vi "StateMachineDAQ-MultiChannel.vi"() -> ()   [LabVIEW 2014]
doc: "Use this template to build a user interface event handler design pattern. Use this pattern for dialog boxes and other user interfaces. You also can create and execute user-defined events that the VI can handle the same way as user interface events."
uses:
  subVIs/StateMachineDAQState.ctl
  <vilib>/Utility/error.llb/DialogType.ctl
  <vilib>/DAQmx/create/channels.llb/DAQmx Create Channel (AI-Voltage-Basic).vi
  <vilib>/DAQmx/configure/timing.llb/DAQmx Timing (Sample Clock).vi
  <vilib>/DAQmx/read.llb/DAQmx Read (Analog 1D Wfm NChan NSamp).vi
  <resource>/objmgr/daqmx.rc
panel:
  in  "File Path":path
  in  "Acquire Data":bool
  in  "Log Data":bool
  in  "File Comment":string
  in  "DAQ Parameters":T1={"rate"=1000.0, "read period"=0.5, "Channels"=[]} {"Channels"."minimum value" format="%0.2f"; "Channels"."maximum value" format="%0.2f"; "read period" format="%0.2f"; "rate" format="%0.2f"}
  out "Waveform Chart":waveform(dbl)[](graph)
  in  "quit":bool
  # "Hz"
  # "s"
  # "V"
  # "V"
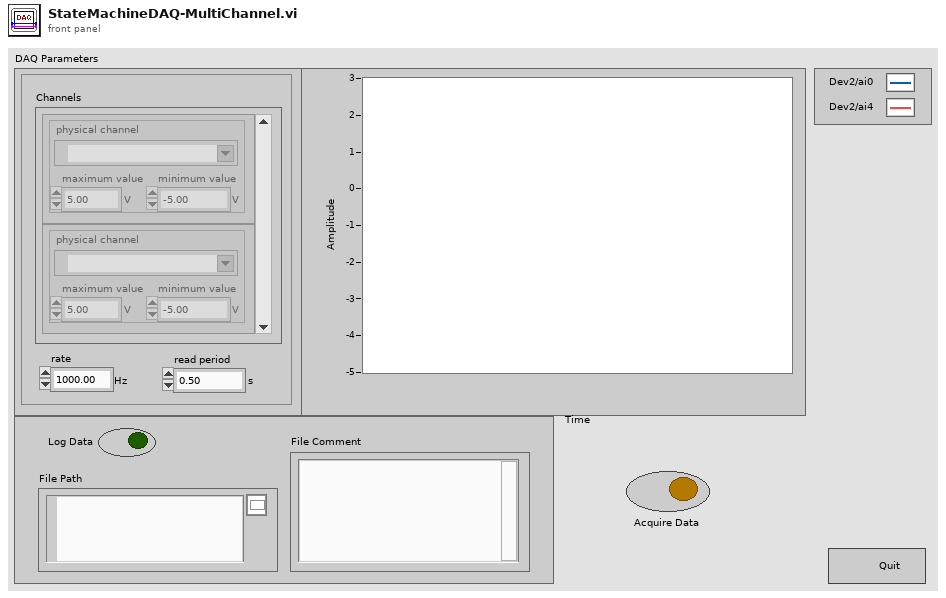
[diagram p1: front panel]
types:
  T1 = cluster{"rate":dbl, "read period":dbl, "Channels":cluster{"physical channel":tag, "maximum value":dbl, "minimum value":dbl}[]}
  T2 = typedef "StateMachineDAQState.ctl" = enum16{"Init", "Idle", "CheckError", "Finalize", "ConfigDAQ", "StartDAQ", "AcquireAndLog", "StopDAQ", "ClearDAQ", "OpenFile", "CloseFile", "Process 1"}
  T3 = typedef "DialogType.ctl" = u16
  T4 = cluster{"physical channel":tag, "maximum value":dbl, "minimum value":dbl}[]
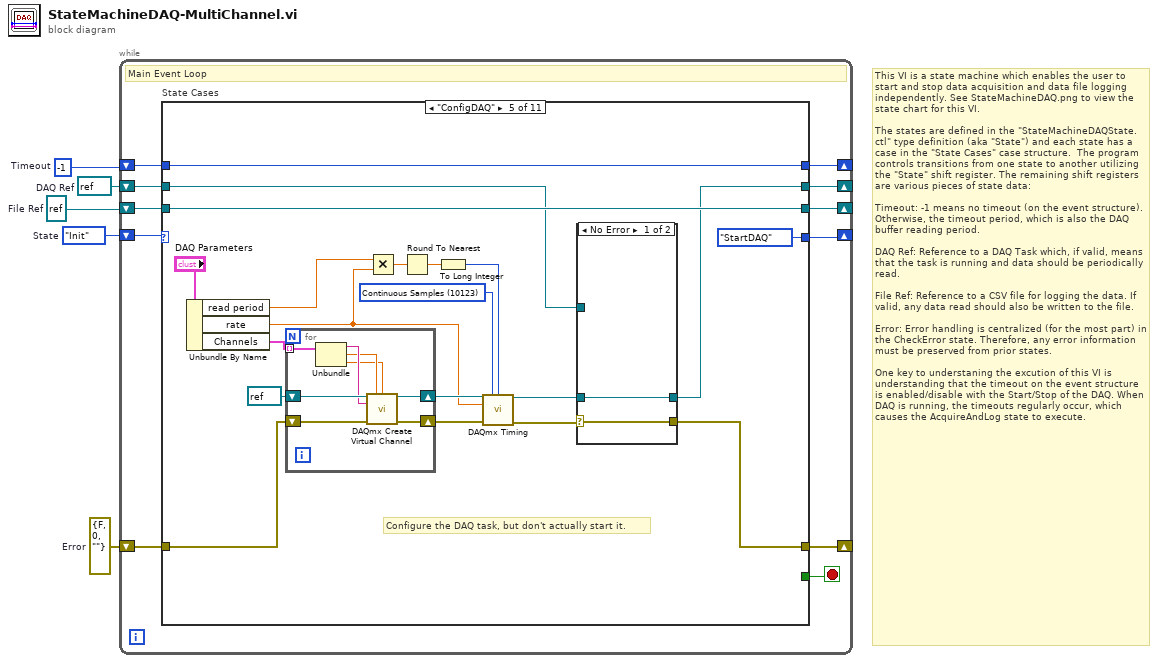
[diagram p0: block diagram]
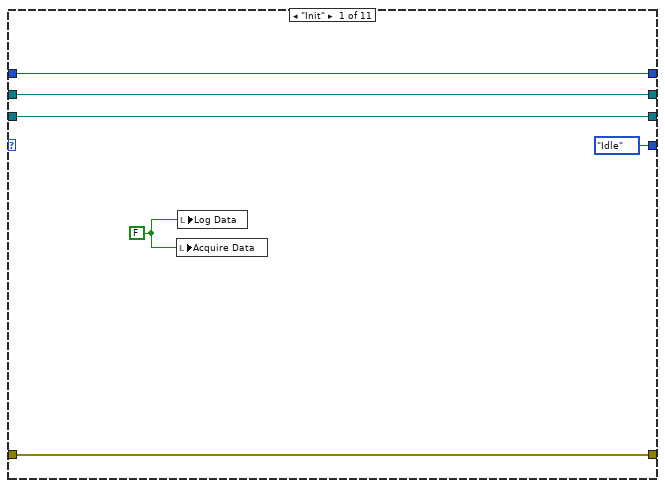
[diagram p2: hidden frame]
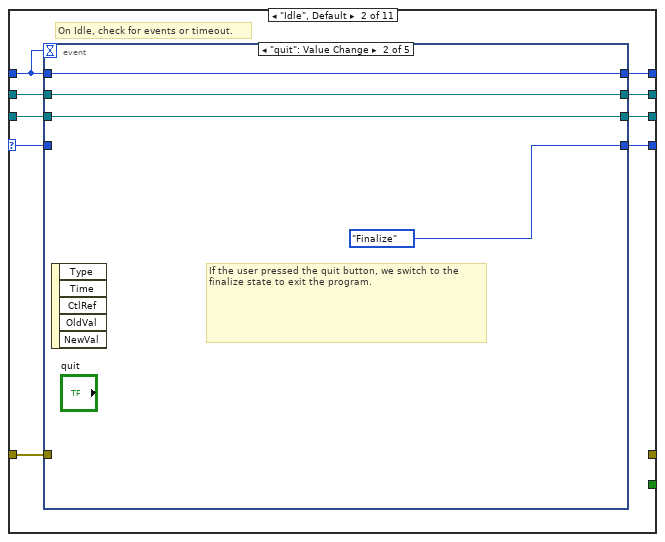
[diagram p3: hidden frame]
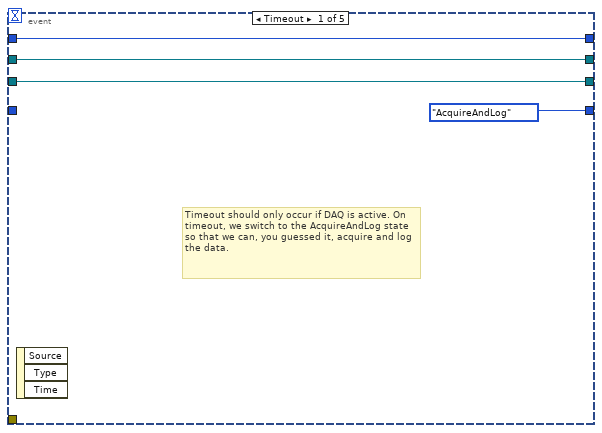
[diagram p4: hidden frame]
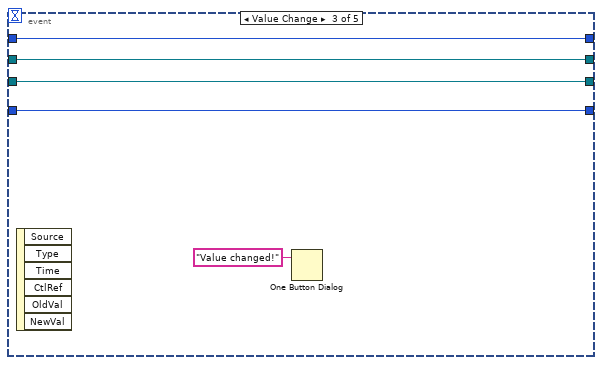
[diagram p5: hidden frame]
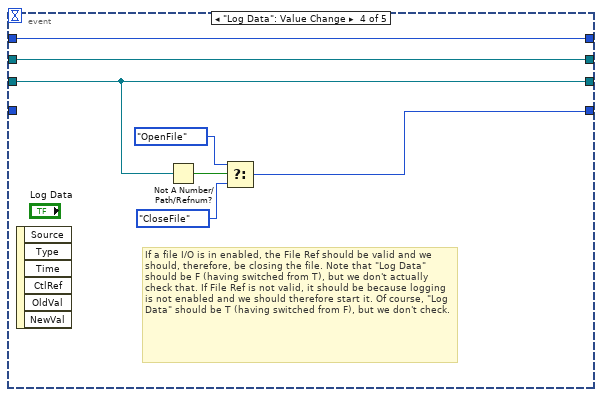
[diagram p6: hidden frame]
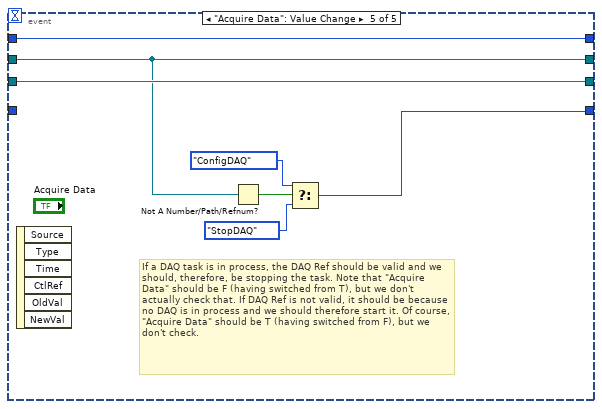
[diagram p7: hidden frame]
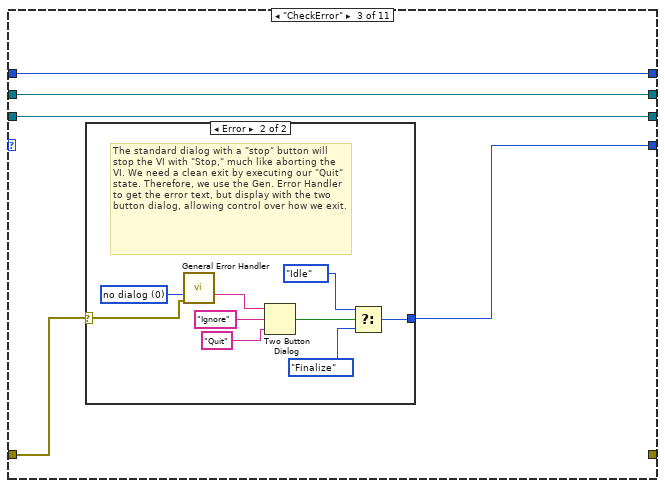
[diagram p8: hidden frame]
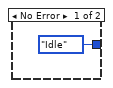
[diagram p9: hidden frame]
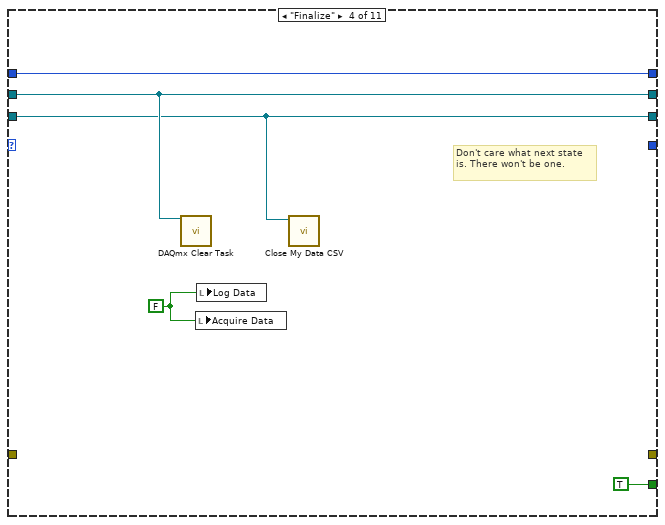
[diagram p10: hidden frame]
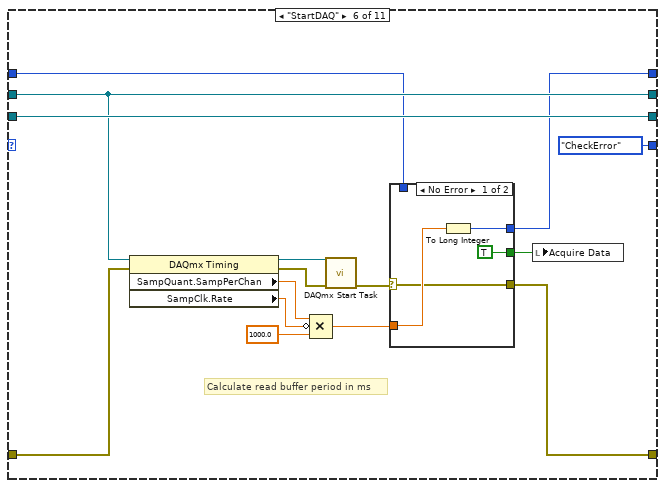
[diagram p12: hidden frame]
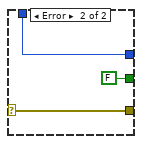
[diagram p13: hidden frame]
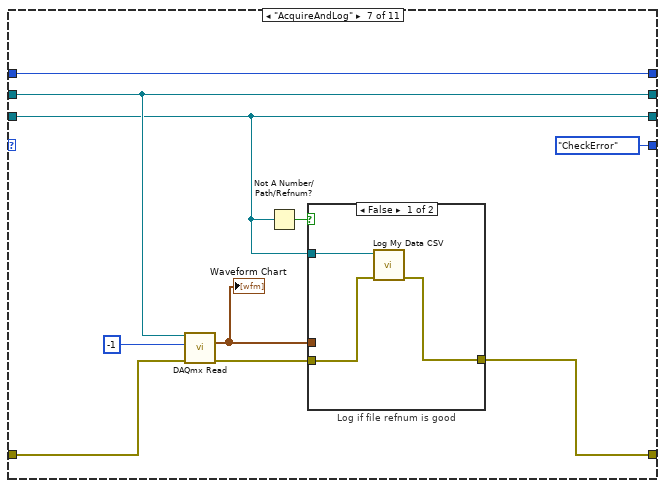
[diagram p14: hidden frame]
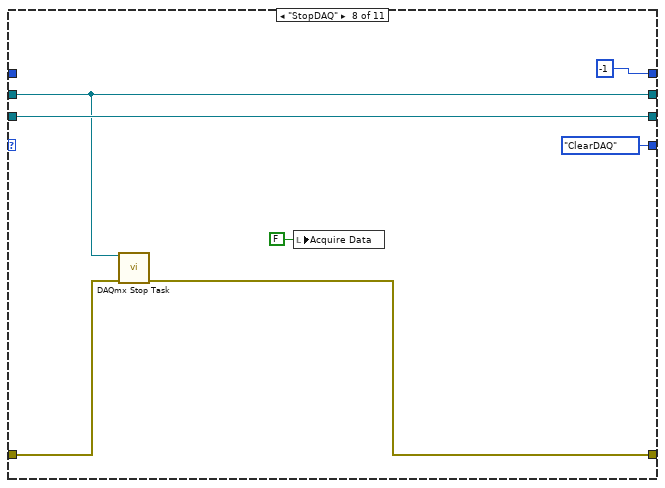
[diagram p16: hidden frame]
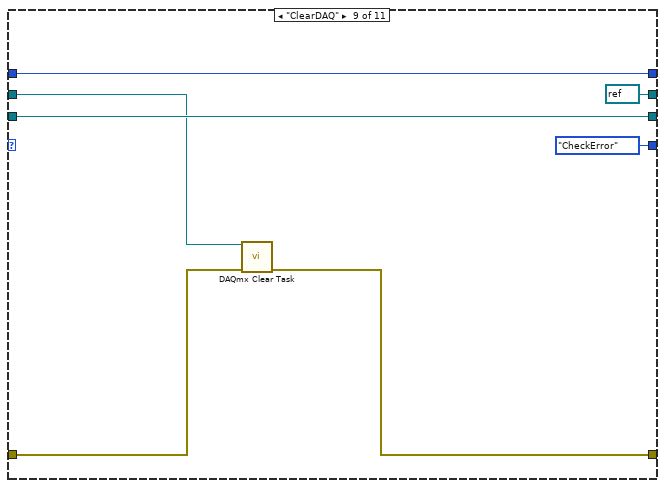
[diagram p17: hidden frame]
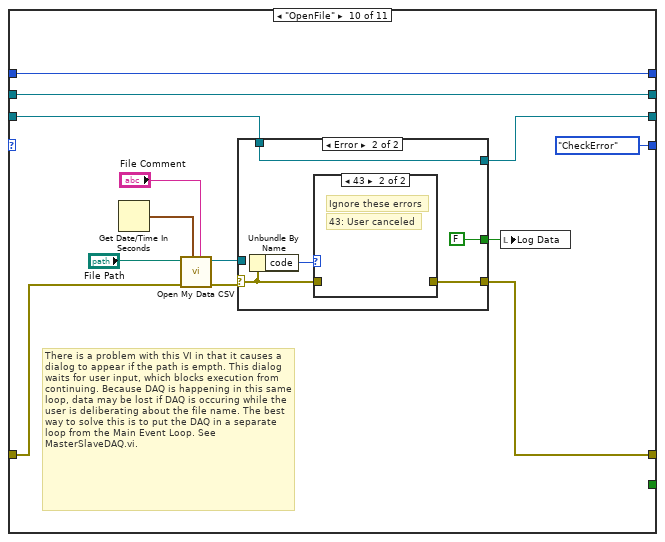
[diagram p18: hidden frame]
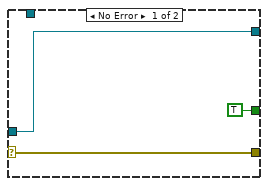
[diagram p19: hidden frame]
diagram:
  w1 = errorcluster {"status"=FALSE, "code"=0, "source"=""}  # Error
  w2 = refnum<file> refnum  # File Ref
  w3 = refnum<k21> refnum  # DAQ Ref
  w4 = StateMachineDAQState."Init"  # State
  w5 = -1  # Timeout
  # "This VI is a state machine which enables the user to start and stop data acquisition and data file logging independently. See StateMachineDAQ.png to view the state chart for this VI.\n\nThe states are defined in the \"StateMachineDAQState.ctl\" type definition (aka \"State\") and each state has a case in the \"State Cases\" case structure.  The program controls transitions from one state to another utilizing the \"State\" shift register. The remaining shift registers are various pieces of state data:\n\nTimeout: -1 means no timeout (on the event structure). Otherwise, the timeout period, which is also the DAQ buffer reading period.\n\nDAQ Ref: Reference to a DAQ Task which, if valid, means that the task is running and data should be periodically read.\n\nFile Ref: Reference to a CSV file for logging the data. If valid, any data read should also be written to the file.\n\nError: Error handling is centralized (for the most part) in the CheckError state. Therefore, any error information must be preserved from prior states.\n\nOne key to understaning the excution of this VI is understanding that the timeout on the event structure is enabled/disable with the Start/Stop of the DAQ. When DAQ is running, the timeouts regularly occur, which causes the AcquireAndLog state to execute."
  n1 = while {
    shift-right: [w15] -> _
    shift-left: w5 -> [w16]
    shift-right: [w13] -> _
    shift-left: w4 -> [w14]
    shift-right: [w12] -> _
    shift-left: w3 -> [w11]
    shift-right: [w10] -> _
    shift-left: w2 -> [w9]
    shift-right: [w8] -> _
    shift-left: w1 -> [w7]
    stop <- w6 stop-if-true
    # "Main Event Loop"
    n2 = case "State Cases" shown="\"ConfigDAQ\"" w14 {
      selector: w14 -> [_ w29 _ _ _ _ _ _ _ _ _]
      tunnel: w16 -> [w22 w31 w63 w78 w86 w120 w139 _ w160 w173 w190]
      tunnel: [w22 w30 w63 w78 w86 w119 w139 -1 ("Timeout") w160 w173 w190] -> w15
      tunnel: [StateMachineDAQState."Idle" ("State") w28 w60 _ StateMachineDAQState."StartDAQ" ("State") StateMachineDAQState."CheckError" ("State") StateMachineDAQState."CheckError" ("State") StateMachineDAQState."ClearDAQ" ("State") StateMachineDAQState."CheckError" ("State") StateMachineDAQState."CheckError" ("State") StateMachineDAQState."CheckError" ("State")] -> w13
      tunnel: [w21 w25 w62 w76 w89 w124 w138 w148 refnum<k21> refnum ("DAQ Ref") w172 w189] -> w12
      tunnel: w11 -> [w21 w24 w62 w76 w90 w124 w138 w148 w156 w172 w189]
      tunnel: [w20 w27 w61 w75 w98 w125 w137 w153 w158 w166 w184] -> w10
      tunnel: w9 -> [w20 w26 w61 w75 w98 w125 w137 w153 w158 w161 w188]
      tunnel: [w17 _ _ _ w87 w118 w136 w149 w154 w165 w186] -> w8
      tunnel: w7 -> [w17 w23 w59 _ w81 w115 w134 w147 w155 w162 w183]
      tunnel: [_ _ _ TRUE _ _ _ _ _ _ _] -> w6
      frame "Init" {
        w18 = FALSE
        n3 = local write "Acquire Data"(w18) -> ()
        n4 = local write "Log Data"(w18) -> ()
      }
      frame "Idle", Default {
        # "On Idle, check for events or timeout."
        # "States"
        n5 = event shown="[1] \"quit\": Value Change" {
          selector: _ -> [_ _ _ _ _]
          dyn-events: _ -> [_ _ _ _ _]
          timeout: w31 -> [_ _ _ _ _]
          tunnel: w31 -> [w35 w39 w44 w51 w58]
          tunnel: [w35 w39 w44 w51 w58] -> w30
          tunnel: w29 -> [_ _ w41 _ _]
          tunnel: [StateMachineDAQState."AcquireAndLog" ("State") StateMachineDAQState."Finalize" ("State") w41 w45 w52] -> w28
          tunnel: [w32 w37 w42 w48 w57] -> w27
          tunnel: w26 -> [w32 w37 w42 w48 w57]
          tunnel: [w34 w38 w43 w50 w55] -> w25
          tunnel: w24 -> [w34 w38 w43 w50 w55]
          tunnel: w23 -> [_ _ _ _ _]
          event Timeout {
            # "Timeout should only occur if DAQ is active. On timeout, we switch to the AcquireAndLog state so that we can, you guessed it, acquire and log the data."
            n6 = event-data() -> ()  [unwired: 1 in, 3 out]
          }
          event "quit": Value Change {
            # "If the user pressed the quit button, we switch to the finalize state to exit the program."
            n7 = event-data() -> ()  [unwired: 1 in, 5 out]
          }
          event "DAQ Parameters.Channels": Value Change {
            n8 = event-data() -> ()  [unwired: 1 in, 6 out]
            n9 = One Button Dialog(message="Value changed!") -> ()  [unwired: 1 in, 1 out]
          }
          event "Log Data": Value Change {
            # "If a file I/O is in enabled, the File Ref should be valid and we should, therefore, be closing the file. Note that \"Log Data\" should be F (having switched from T), but we don't actually check that. If File Ref is not valid, it should be because logging is not enabled and we should therefore start it. Of course, \"Log Data\" should be T (having switched from F), but we don't check."
            n10 = event-data() -> ()  [unwired: 1 in, 6 out]
            n11 = Not A Number/Path/Refnum?(number/path/refnum=w48) -> (NaN/Path/Refnum?=w49:bool)
            n12 = Select(t=StateMachineDAQState."OpenFile" ("State"), s=w49, f=StateMachineDAQState."CloseFile" ("State")) -> (s? t:f=w45:T2)
          }
          event "Acquire Data": Value Change {
            # "If a DAQ task is in process, the DAQ Ref should be valid and we should, therefore, be stopping the task. Note that \"Acquire Data\" should be F (having switched from T), but we don't actually check that. If DAQ Ref is not valid, it should be because no DAQ is in process and we should therefore start it. Of course, \"Acquire Data\" should be T (having switched from F), but we don't check."
            n13 = event-data() -> ()  [unwired: 1 in, 6 out]
            n14 = Not A Number/Path/Refnum?(number/path/refnum=w55) -> (NaN/Path/Refnum?=w56:bool)
            n15 = Select(t=StateMachineDAQState."ConfigDAQ" ("State"), s=w56, f=StateMachineDAQState."StopDAQ" ("State")) -> (s? t:f=w52:T2)
          }
        }
      }
      frame "CheckError" {
        n16 = case shown="Error" w59 {
          selector: w59 -> [_ w65]
          tunnel: [StateMachineDAQState."Idle" ("State") w66] -> w60
          frame No Error {
          }
          frame Error {
            w73 = T3 0 items=["no dialog", "OK message", "continue or stop message", "OK message + warnings", "continue/stop + warnings"] ("type of dialog (OK msg:1)")
            # "The standard dialog with a \"stop\" button will stop the VI with \"Stop,\" much like aborting the VI. We need a clean exit by executing our \"Quit\" state. Therefore, we use the Gen. Error Handler to get the error text, but display with the two button dialog, allowing control over how we exit."
            n17 = call <vilib>:"General Error Handler.vi"("type of dialog (OK msg:1)"=w73, "error in (no error)"=w65) -> ("message"=w72:string)  [unwired: 9 in, 4 out]
            n18 = Two Button Dialog(message=w72, 1:"Quit" ("F button name (\"Cancel\")"), 2:"Ignore" ("T button name (\"OK\")")) -> (T button?=w69:bool)
            n19 = Select(t=StateMachineDAQState."Idle" ("State"), s=w69, f=StateMachineDAQState."Finalize" ("State")) -> (s? t:f=w66:T2)
          }
        }
      }
      frame "Finalize" {
        w74 = FALSE
        # "Don't care what next state is. There won't be one."
        n20 = call <vilib>:"DAQmx Clear Task.vi"("task in"=w76) -> ()  [unwired: 14 in, 1 out]
        n21 = local write "Acquire Data"(w74) -> ()
        n22 = local write "Log Data"(w74) -> ()
        n23 = call "Close My Data CSV.vi"("file refnum"=w75) -> ()  [unwired: 10 in, 1 out]
      }
      frame "ConfigDAQ" {
        w95 = 10123 items=["Finite Samples"=10178, "Continuous Samples"=10123, "Hardware Timed Single Point"=12522] ("sample mode")
        # "Configure the DAQ task, but don't actually start it."
        n24 = Unbundle By Name("DAQ Parameters") -> ("read period"=w83:dbl, "rate"=w82:dbl, "Channels"=w79:T4)
        n25 = for {
          shift-right: [w105] -> w96
          shift-left: w81 -> [w104]
          shift-right: [w106] -> w97
          shift-left: refnum<k21> refnum ("task out") -> [w102]
          tunnel: w79 -> [w103] mode=indexing
          n26 = Unbundle(w103) -> ("physical channel"=w101:tag, "maximum value"=w100:dbl, "minimum value"=w99:dbl)
          n27 = call-poly <vilib>:"DAQmx Create Virtual Channel.vi"("task in"=w102, "maximum value"=w100, "minimum value"=w99, "physical channels"=w101, "error in"=w104) -> ("task out"=w106:refnum<k21>, "error out"=w105:errorcluster)  [unwired: 9 in]
        }
        n28 = Multiply(x=w83, y=w82) -> (x*y=w94:dbl)
        n29 = Round To Nearest(number=w94) -> (nearest integer value=w93:dbl)
        n30 = To Long Integer(number=w93) -> (32bit integer=w92:i32)
        n31 = call-poly <vilib>:"DAQmx Timing.vi"("task/channels in"=w97, "sample mode"=w95, "samples per channel"=w92, "rate"=w82, "error in"=w96) -> ("task out"=w88:refnum<k21>, "error out"=w91:errorcluster)  [unwired: 9 in]
        n32 = case shown="No Error" w91 {
          selector: w91 -> [w107 w110]
          tunnel: w90 -> [_ w109]
          tunnel: [w108 w109] -> w89
          tunnel: w88 -> [w108 _]
          tunnel: [w107 w110] -> w87
          frame No Error {
          }
          frame Error {
          }
        }
      }
      frame "StartDAQ" {
        # "Calculate read buffer period in ms"
        n33 = property class="DAQmx Timing"(reference=w124, error in=w115) -> (reference out=w123:refnum<k21>, error out=w122:errorcluster, "SampQuant.SampPerChan"=w114:dbl, "SampClk.Rate"=w113:dbl)
        n34 = Compound Arithmetic op=MULTIPLY(w114, invert w113, 1000.0 ("value")) -> (w111:dbl)
        n35 = call <vilib>:"DAQmx Start Task.vi"("task/channels in"=w123, "error in"=w122) -> ("error out"=w121:errorcluster)  [unwired: 12 in, 1 out]
        n36 = case shown="No Error" w121 {
          selector: w121 -> [w127 w131]
          tunnel: w111 -> [w129 _]
          tunnel: w120 -> [_ w132]
          tunnel: [w128 w132] -> w119
          tunnel: [w127 w131] -> w118
          tunnel: [TRUE FALSE] -> w116
          frame No Error {
            n37 = To Long Integer(number=w129) -> (32bit integer=w128:i32)
          }
          frame Error {
          }
        }
        n38 = local write "Acquire Data"(w116) -> ()
      }
      frame "AcquireAndLog" {
        n39 = call-poly <vilib>:"DAQmx Read.vi"("task/channels in"=w138, "number of samples per channel"=-1, "error in"=w134) -> ("data"=w133:waveform(dbl)[], "error out"=w140:errorcluster)  [unwired: 10 in, 1 out]
        "Waveform Chart" <- w133
        n40 = Not A Number/Path/Refnum?(number/path/refnum=w137) -> (NaN/Path/Refnum?=w141:bool)
        n41 = case "Log if file refnum is good" shown="False" w141 {
          tunnel: w140 -> [w144 w146]
          tunnel: w137 -> [w145 _]
          tunnel: w133 -> [_ _]
          tunnel: [w143 w146] -> w136
          frame False {
            n42 = call "Log My Data CSV.vi"("error in"=w144, "file refnum"=w145) -> ("error out"=w143:errorcluster)  [unwired: 8 in, 1 out]
          }
          frame True {
          }
        }
      }
      frame "StopDAQ" {
        n43 = call <vilib>:"DAQmx Stop Task.vi"("task/channels in"=w148, "error in"=w147) -> ("error out"=w149:errorcluster)  [unwired: 12 in, 1 out]
        n44 = local write "Acquire Data"(FALSE ("Acquire Data")) -> ()
      }
      frame "ClearDAQ" {
        n45 = call <vilib>:"DAQmx Clear Task.vi"("task in"=w156, "error in"=w155) -> ("error out"=w154:errorcluster)  [unwired: 13 in]
      }
      frame "OpenFile" {
        # "There is a problem with this VI in that it causes a dialog to appear if the path is empth. This dialog waits for user input, which blocks execution from continuing. Because DAQ is happening in this same loop, data may be lost if DAQ is occuring while the user is deliberating about the file name. The best way to solve this is to put the DAQ in a separate loop from the Main Event Loop. See MasterSlaveDAQ.vi."
        n46 = Get Date/Time In Seconds() -> (seconds since 1Jan1904=w171:timestamp)
        n47 = call "Open My Data CSV.vi"("Comment"="File Comment", "Time Stamp"=w171, "error in"=w162, "file path"="File Path") -> ("error out"=w168:errorcluster, "refnum out"=w167:refnum<file>)  [unwired: 6 in]
        n48 = case shown="Error" w168 {
          selector: w168 -> [w175 w178]
          tunnel: [w176 w180] -> w166
          tunnel: w167 -> [w176 _]
          tunnel: [w175 w177] -> w165
          tunnel: [TRUE ("Log Data") FALSE ("Log Data")] -> w164
          tunnel: w161 -> [_ w180]
          frame No Error {
          }
          frame Error {
            n49 = Unbundle By Name(w178) -> ("code"=w179:i32)
            n50 = case shown="43" w179 {
              tunnel: w178 -> [w182 _]
              tunnel: [w182 _] -> w177
              frame 1, Default {
                # "Process these errors"
              }
              frame 43 {
                # "43: User canceled"
                # "Ignore these errors"
              }
            }
          }
        }
        n51 = local write "Log Data"(w164) -> ()
      }
      frame "CloseFile" {
        w184 = refnum<file> refnum  # File Ref
        n52 = call "Close My Data CSV.vi"("error in"=w183, "file refnum"=w188) -> ("error out"=w186:errorcluster)  [unwired: 9 in]
        n53 = local write "Log Data"(FALSE ("Log Data")) -> ()
      }
    }
  }
